vi "Update Cage Layout.vi"(8 "error in (no error)":errorcluster, 9 "Pixel <> Zone":T1, 10 "Cage Diagram ref":T2) -> (0 "error out":errorcluster)   [LabVIEW 2018, in "Tracker Main.lvlib"]
doc: "Updates Cage layout when it comes from the Cage Diagram module.\n_____\nCreated using Delacor QMH Event Scripter 4.2.1.88."
uses:
  Tracker Main.lvlib
  <vilib>/vision/Image Controls.llb/IMAQ Image.ctl
  SubVi's/Controls/CTL_Pixel_to_Zone_array.ctl
  Update Cage Layout Argument--cluster.ctl
  Common_Resources.lvlib
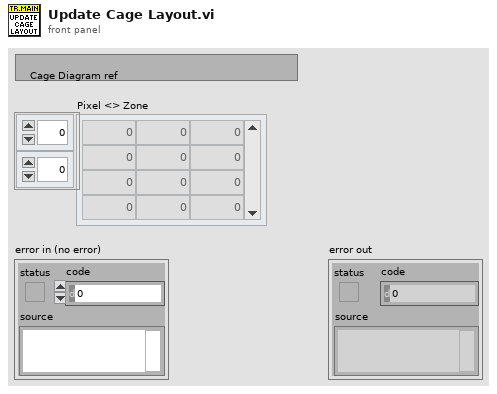
[diagram p1: front panel]
types:
  T1 = typedef "Common_Resources.lvlib/CTL_Pixel_to_Zone_array.ctl" = i8[][]
  T2 = typedef "IMAQ Image.ctl" = refnum<image>
  T3 = typedef "Tracker Main.lvlib/Update Cage Layout Argument--cluster.ctl" = cluster{"Cage Diagram ref":T2, "Pixel <> Zone":T1}
  T4 = typedef "Tracker Main.lvlib/Request Events--cluster.ctl" = cluster{"Stop Module":refnum<user-event>, "Show Panel":refnum<user-event>, "Hide Panel":refnum<user-event>, "Get Module Execution Status":refnum<user-event>, "Show Diagram":refnum<user-event>, "SW Init":refnum<user-event>, "Prepare to Exit":refnum<user-event>, "Update Status and History":refnum<user-event>, "Update Interface":refnum<user-event>, "HW Init":refnum<user-event>, "Load Minimal Set of Modules":refnum<user-event>, "Update Cage Layout":refnum<user-event>}
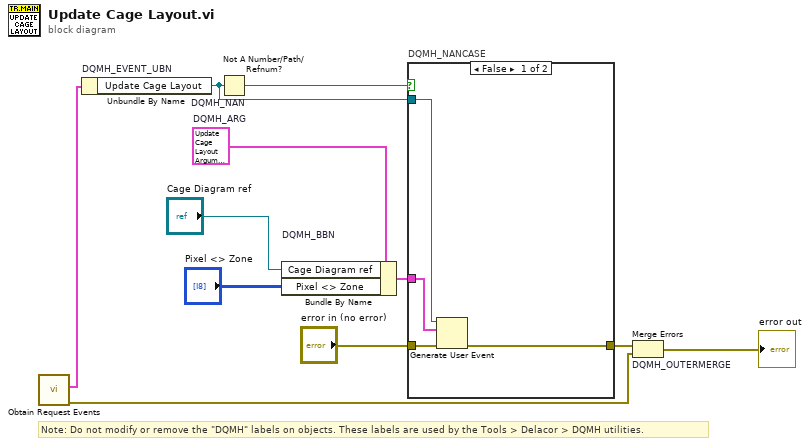
[diagram p0: block diagram]
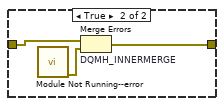
[diagram p2: hidden frame]
diagram:
  w5 = T3 {"Cage Diagram ref"=refnum, "Pixel <> Zone"=[]}  # DQMH_ARG
  # "Note: Do not modify or remove the \"DQMH\" labels on objects. These labels are used by the Tools > Delacor > DQMH utilities."
  n1 = call "Obtain Request Events.vi"() -> ("error out"=w2:errorcluster, "Tracker Main Request Events"=w1:T4)  [unwired: 10 in]
  n2 = Unbundle By Name "DQMH_EVENT_UBN"(w1) -> ("Update Cage Layout"=w7:refnum<user-event>)
  n3 = Not A Number/Path/Refnum? "DQMH_NAN"(number/path/refnum=w7) -> (NaN/Path/Refnum?=w8:bool)
  n4 = Bundle By Name "DQMH_BBN"(cluster=w5, "Cage Diagram ref"="Cage Diagram ref", "Pixel <> Zone"="Pixel <> Zone") -> (w9:T3)
  n5 = case "DQMH_NANCASE" shown="False" w8 {
    tunnel: "error in (no error)" -> [w15 w18]
    tunnel: [w14 w17] -> w6
    tunnel: w7 -> [w13 _]
    tunnel: w9 -> [w12 _]
    frame False {
      n6 = Generate User Event(user event=w13, event data cluster=w12, error in=w15) -> (error out=w14:errorcluster)  [unwired: 1 in, 1 out]
    }
    frame True {
      n7 = call "Module Not Running--error.vi"() -> ("error out"=w16:errorcluster)  [unwired: 11 in]
      n8 = Merge Errors "DQMH_INNERMERGE"(w18, w16) -> (w17:errorcluster)
    }
  }
  n9 = Merge Errors "DQMH_OUTERMERGE"(w6, w2) -> (→"error out":errorcluster)
